vi "test_display_image.vi"() -> ()   [LabVIEW 2019]
panel:
  in  "display_2":bool
  in  "display_1":bool
  in  "stop":bool
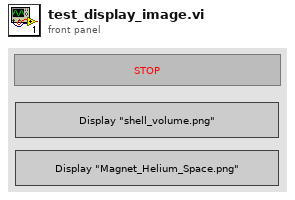
[diagram p1: front panel]
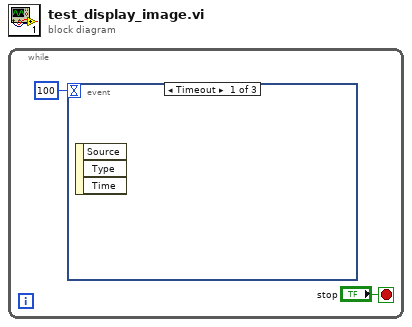
[diagram p0: block diagram]
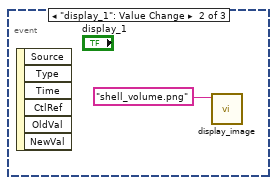
[diagram p2: hidden frame]
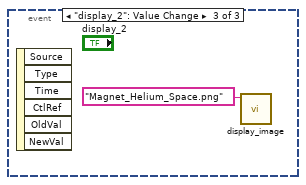
[diagram p3: hidden frame]
diagram:
  n1 = while {
    stop <- "stop" stop-if-true
    n2 = event shown="[0] Timeout" {
      selector: _ -> [_ _ _]
      dyn-events: _ -> [_ _ _]
      timeout: 100 -> [_ _ _]
      event Timeout {
        n3 = event-data() -> ()  [unwired: 1 in, 3 out]
      }
      event "display_1": Value Change {
        n4 = event-data() -> ()  [unwired: 1 in, 6 out]
        n5 = call "display_image.vi"("file_name"="shell_volume.png") -> ()  [unwired: 8 in, 3 out]
      }
      event "display_2": Value Change {
        n6 = event-data() -> ()  [unwired: 1 in, 6 out]
        n7 = call "display_image.vi"("file_name"="Magnet_Helium_Space.png") -> ()  [unwired: 8 in, 3 out]
      }
    }
  }
